vi "PIDController_Calculate_PV.vi"(10 "PV":dbl, 11 "in PID_CONTROLLER":T1={"Kp"=0.0, "Ki"=0.0, "Kd"=0.0, "Period"=0.0, "Max_Integral"=0.0, "Min_Integral"=0.0, "Max_Input"=0.0, "Min_Input"=0.0, "Continuous"=FALSE, "PositionError"=0.0, "VelocityError"=0.0, "PrevError"=0.0, "TotalError"=0.0, "PositionTolerance"=0.0, "VelocityTolerance"=0.0, "SetPoint"=0.0, "Kf"=0.0, "Prev_Deriv"=0.0, "Prev_Deriv 2"=0.0, "DerivativeFilter"=FALSE, "Min_Output"=-9.99e+35, "Max_Output"=9.9e+35, "Prev_F_P"=0.0, "Prev_F_P_2"=0.0, "AntiWindupActive"=FALSE, "Measurement"=0.0} {"Measurement" format="%16_6e"; "Prev_F_P_2" format="%16_6e"; "Prev_F_P" format="%16_6e"; "Max_Output" format="%16_6e"; "Min_Output" format="%16_6e"; "Prev_Deriv 2" format="%16_6e"; "Prev_Deriv" format="%16_6e"; "Kf" format="%16_6e"; "SetPoint" format="%16_6e"; "VelocityTolerance" format="%16_6e"; "PositionTolerance" format="%16_6e"; "TotalError" format="%16_6e"; "PrevError" format="%16_6e"; "VelocityError" format="%16_6e"; "PositionError" format="%16_6e"; "Min_Input" format="%16_6e"; "Max_Input" format="%16_6e"; "Min_Integral" format="%16_6e"; "Max_Integral" format="%16_6e"; "Period" format="%16_6e"; "Kd" format="%16_6e"; "Ki" format="%16_6e"; "Kp" format="%16_6e"}) -> (1 "ControlOutput":dbl, 3 "out PID_CONTROLLER":T1={"Kp"=0.0, "Ki"=0.0, "Kd"=0.0, "Period"=0.0, "Max_Integral"=0.0, "Min_Integral"=0.0, "Max_Input"=0.0, "Min_Input"=0.0, "Continuous"=FALSE, "PositionError"=0.0, "VelocityError"=0.0, "PrevError"=0.0, "TotalError"=0.0, "PositionTolerance"=0.0, "VelocityTolerance"=0.0, "SetPoint"=0.0, "Kf"=0.0, "Prev_Deriv"=0.0, "Prev_Deriv 2"=0.0, "DerivativeFilter"=FALSE, "Min_Output"=-9.99e+35, "Max_Output"=9.9e+35, "Prev_F_P"=0.0, "Prev_F_P_2"=0.0, "AntiWindupActive"=FALSE, "Measurement"=0.0} {"Measurement" format="%16_6e"; "Prev_F_P_2" format="%16_6e"; "Prev_F_P" format="%16_6e"; "Max_Output" format="%16_6e"; "Min_Output" format="%16_6e"; "Prev_Deriv 2" format="%16_6e"; "Prev_Deriv" format="%16_6e"; "Kf" format="%16_6e"; "SetPoint" format="%16_6e"; "VelocityTolerance" format="%16_6e"; "PositionTolerance" format="%16_6e"; "TotalError" format="%16_6e"; "PrevError" format="%16_6e"; "VelocityError" format="%16_6e"; "PositionError" format="%16_6e"; "Min_Input" format="%16_6e"; "Max_Input" format="%16_6e"; "Min_Integral" format="%16_6e"; "Max_Integral" format="%16_6e"; "Period" format="%16_6e"; "Kd" format="%16_6e"; "Ki" format="%16_6e"; "Kp" format="%16_6e"})   [LabVIEW 2019, in "Trajectory_Library.lvlib"]
doc: "Returns the next output of the PID controller. The saved setpoint (SP) in the PID_Controller data structure is used.\n \nInputs:\n - PID_Controller -- PID_Controller data cluster\n - PV-measurement -- The current measurement of the process variable. (PV)\n\nOutputs:\n - PID_Controller -- Updated PID_Controller data cluster\n - CO-ControlOutput -- Controller output (CO)"
uses:
  Trajectory_Library.lvlib
  PID_CONTROLLER.ctl
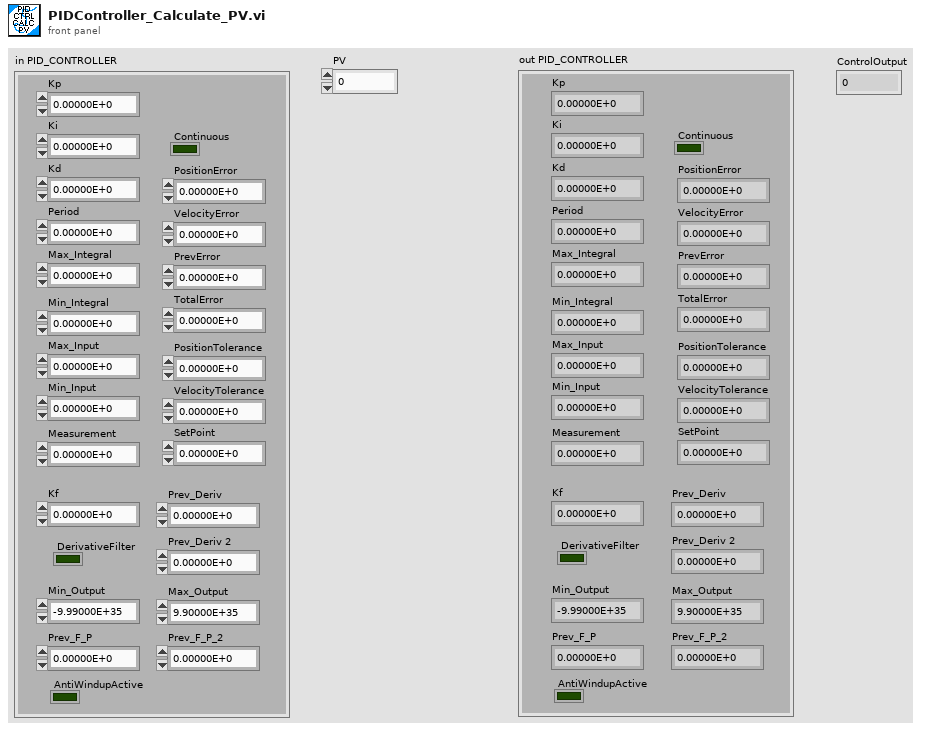
[diagram p1: front panel]
types:
  T1 = typedef "Trajectory_Library.lvlib/PID_CONTROLLER.ctl" = cluster{"Kp":dbl, "Ki":dbl, "Kd":dbl, "Period":dbl, "Max_Integral":dbl, "Min_Integral":dbl, "Max_Input":dbl, "Min_Input":dbl, "Continuous":bool, "PositionError":dbl, "VelocityError":dbl, "PrevError":dbl, "TotalError":dbl, "PositionTolerance":dbl, "VelocityTolerance":dbl, "SetPoint":dbl, "Kf":dbl, "Prev_Deriv":dbl, "Prev_Deriv 2":dbl, "DerivativeFilter":bool, "Min_Output":dbl, "Max_Output":dbl, "Prev_F_P":dbl, "Prev_F_P_2":dbl, "AntiWindupActive":bool, "Measurement":dbl}
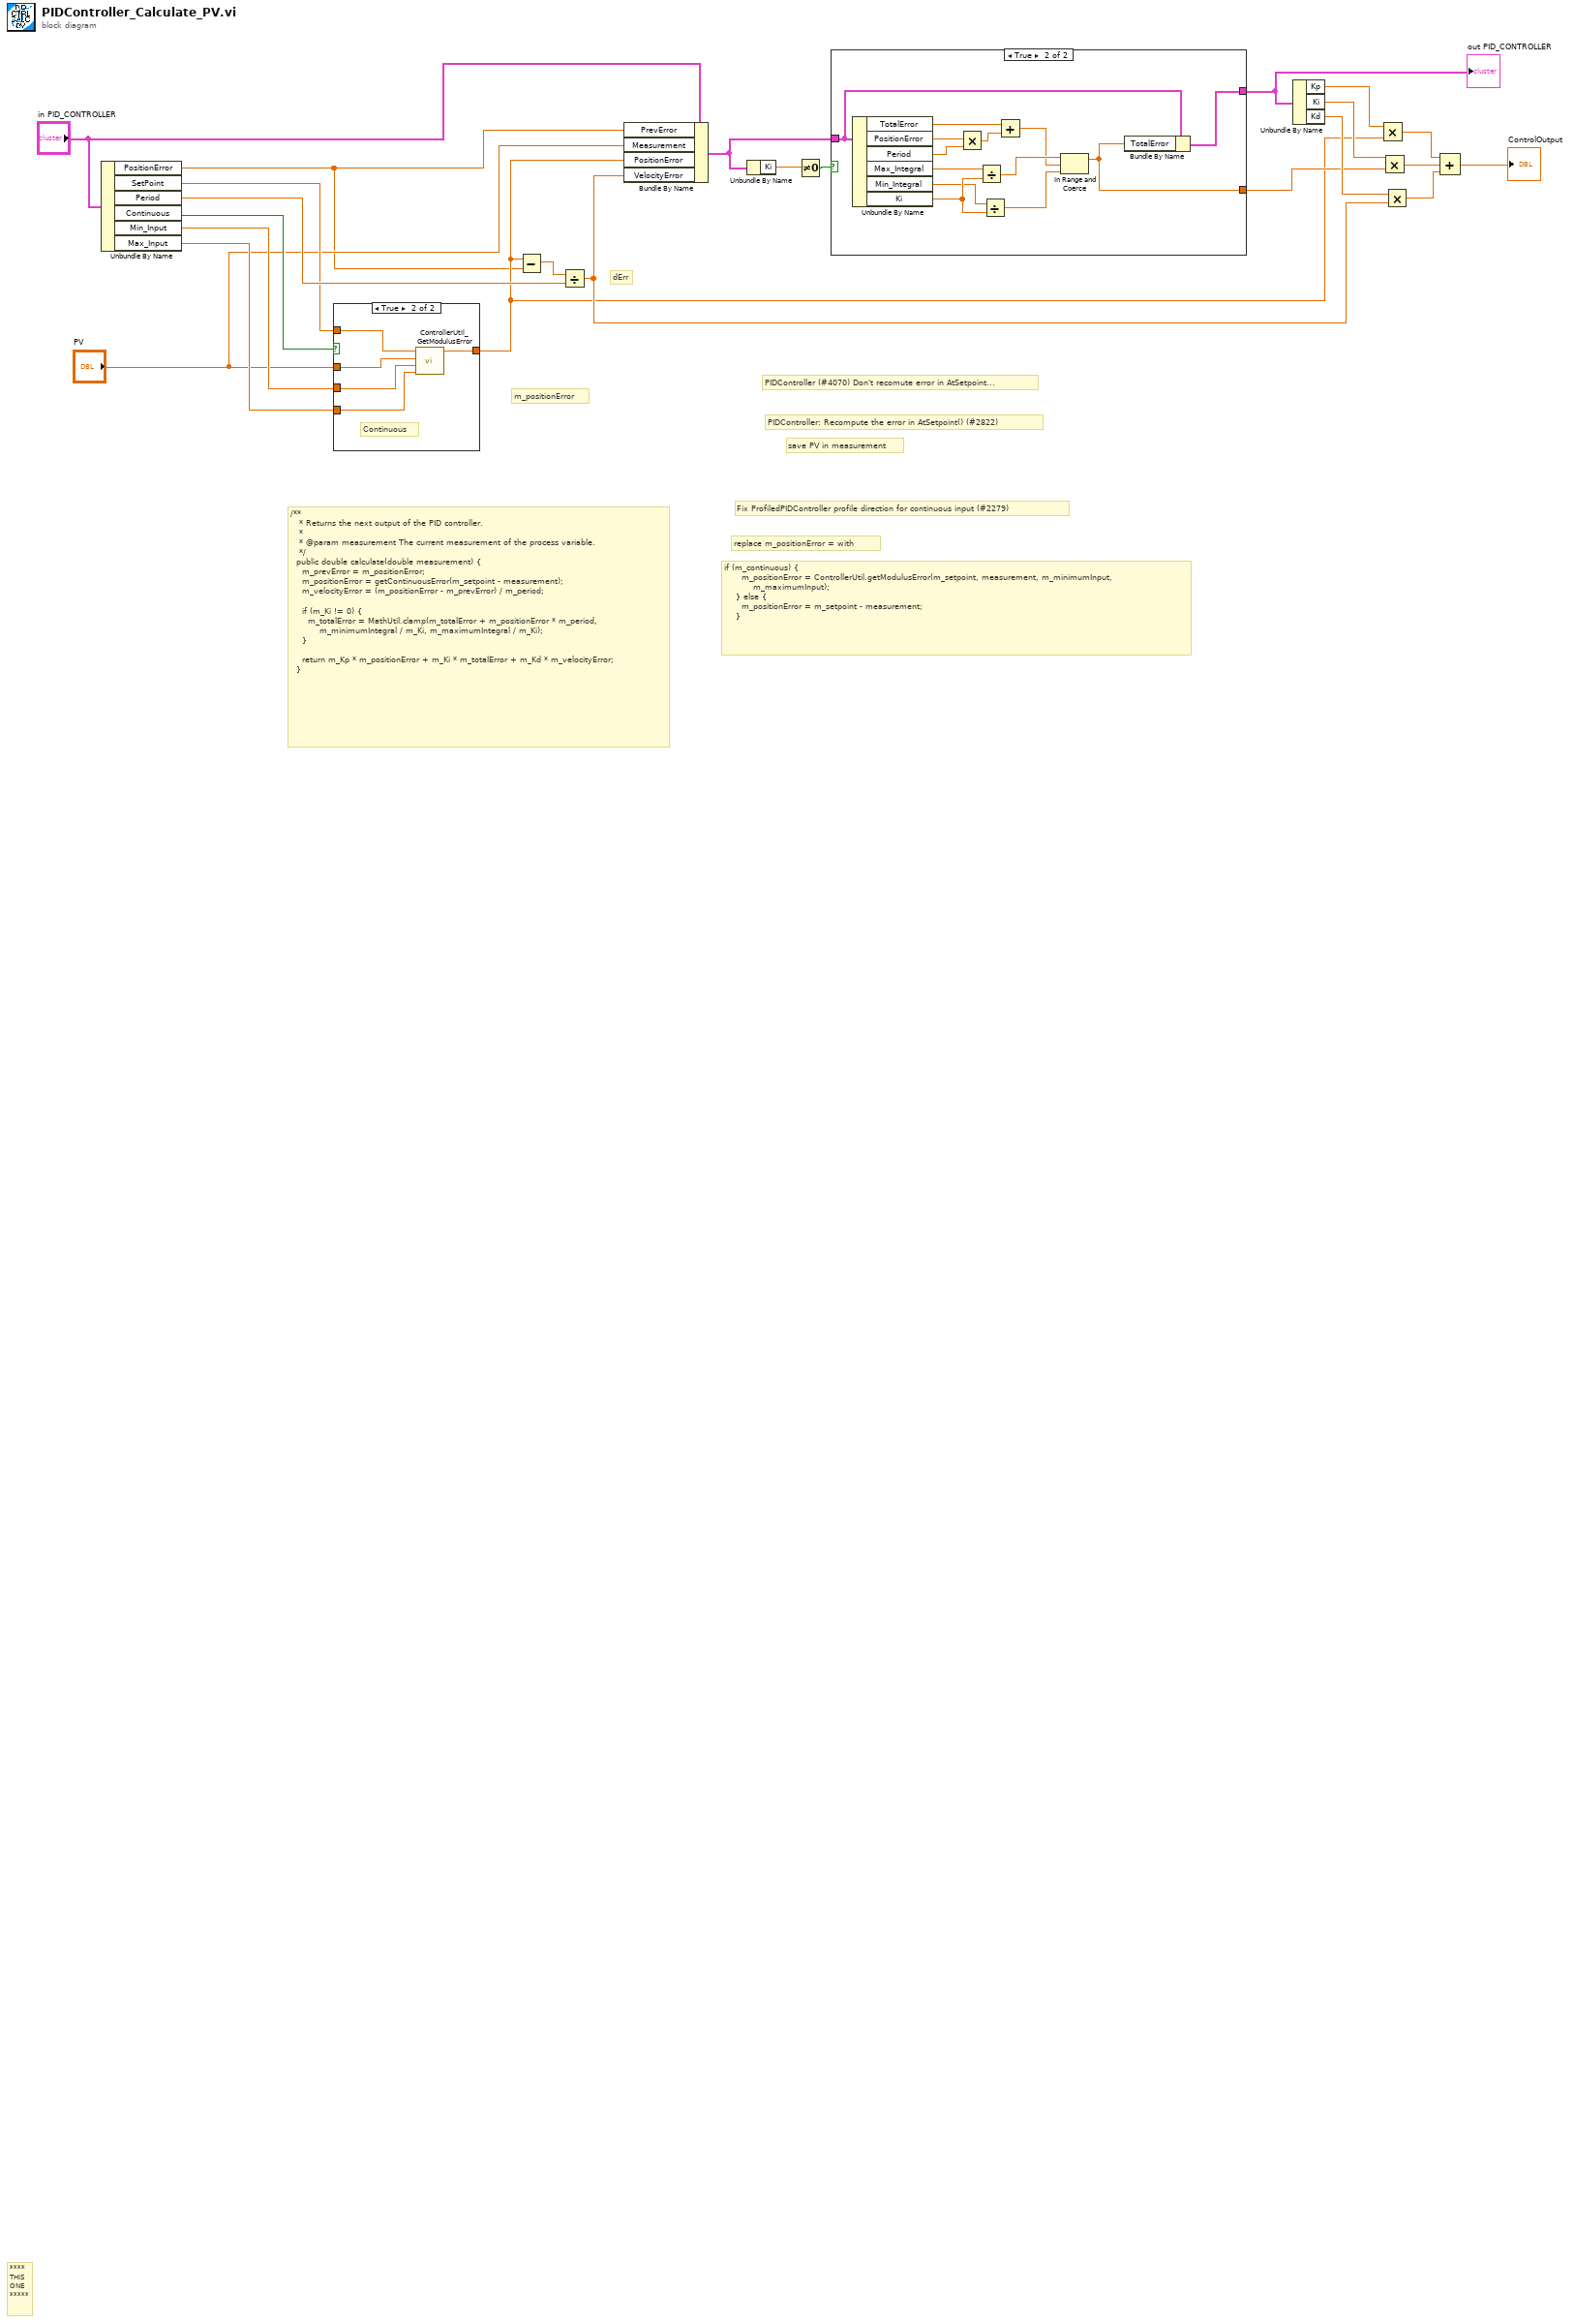
[diagram p0: block diagram]
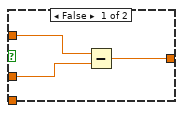
[diagram p2: hidden frame]
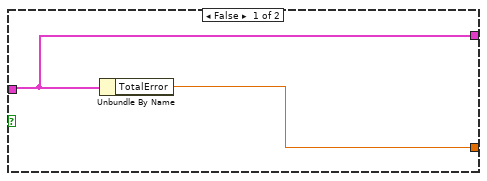
[diagram p3: hidden frame]
diagram:
  # "PIDController (#4070) Don't recomute error in AtSetpoint..."
  # "dErr"
  # "save PV in measurement"
  # "PIDController: Recompute the error in AtSetpoint() (#2822)"
  # "m_positionError"
  # "Fix ProfiledPIDController profile direction for continuous input (#2279)"
  # "replace m_positionError = with"
  # "if (m_continuous) {\n      m_positionError = ControllerUtil.getModulusError(m_setpoint, measurement, m_minimumInput,\n          m_maximumInput);\n    } else {\n      m_positionError = m_setpoint - measurement;\n    }"
  # "/**\n   * Returns the next output of the PID controller.\n   *\n   * @param measurement The current measurement of the process variable.\n   */\n  public double calculate(double measurement) {\n    m_prevError = m_positionError;\n    m_positionError = getContinuousError(m_setpoint - measurement);\n    m_velocityError = (m_positionError - m_prevError) / m_period;\n\n    if (m_Ki != 0) {\n      m_totalError = MathUtil.clamp(m_totalError + m_positionError * m_period,\n          m_minimumIntegral / m_Ki, m_maximumIntegral / m_Ki);\n    }\n\n    return m_Kp * m_positionError + m_Ki * m_totalError + m_Kd * m_velocityError;\n  }"
  # "****\nTHIS\nONE\n*****"
  n1 = Unbundle By Name("in PID_CONTROLLER") -> ("PositionError"=w2:dbl, "SetPoint"=w8:dbl, "Period"=w22:dbl, "Continuous"=w9:bool, "Min_Input"=w6:dbl, "Max_Input"=w5:dbl)
  n2 = case shown="True" w9 {
    tunnel: w8 -> [w26 w31]
    tunnel: "PV" -> [w25 w30]
    tunnel: [w24 w27] -> w7
    tunnel: w6 -> [_ w29]
    tunnel: w5 -> [_ w28]
    frame False {
      n3 = Subtract(x=w26, y=w25) -> (x-y=w24:dbl)
    }
    frame True {
      # "Continuous"
      n4 = call "ControllerUtil_GetModulusError.vi"("Maximum_Input"=w28, "Minimum_Input"=w29, "Measurerment(PV)"=w30, "Reference(SP)"=w31) -> ("Error"=w27:dbl)  [unwired: 7 in]
    }
  }
  n5 = Subtract(x=w7, y=w2) -> (x-y=w23:dbl)
  n6 = Divide(x=w23, y=w22) -> (x/y=w10:dbl)
  n7 = Bundle By Name(cluster="in PID_CONTROLLER", "PrevError"=w2, "Measurement"="PV", "PositionError"=w7, "VelocityError"=w10) -> (w3:T1)
  n8 = Unbundle By Name(w3) -> ("Ki"=w21:dbl)
  n9 = Not Equal To 0?(x=w21) -> (x != 0?=w20:bool)
  n10 = case shown="True" w20 {
    tunnel: w3 -> [w32 w36]
    tunnel: [w32 w35] -> w13
    tunnel: [w33 w34] -> w11
    frame False {
      n11 = Unbundle By Name(w32) -> ("TotalError"=w33:dbl)
    }
    frame True {
      n12 = Unbundle By Name(w36) -> ("TotalError"=w45:dbl, "PositionError"=w44:dbl, "Period"=w43:dbl, "Max_Integral"=w41:dbl, "Min_Integral"=w40:dbl, "Ki"=w42:dbl)
      n13 = Multiply(x=w44, y=w43) -> (x*y=w46:dbl)
      n14 = Divide(x=w41, y=w42) -> (x/y=w39:dbl)
      n15 = Divide(x=w40, y=w42) -> (x/y=w38:dbl)
      n16 = Add(x=w45, y=w46) -> (x+y=w37:dbl)
      n17 = In Range and Coerce(upper limit=w39, x=w37, lower limit=w38) -> (coerced(x)=w34:dbl)  [unwired: 1 out]
      n18 = Bundle By Name(cluster=w36, "TotalError"=w34) -> (w35:T1)
    }
  }
  "out PID_CONTROLLER" <- w13
  n19 = Unbundle By Name(w13) -> ("Kp"=w16:dbl, "Ki"=w15:dbl, "Kd"=w14:dbl)
  n20 = Multiply(x=w16, y=w7) -> (x*y=w19:dbl)
  n21 = Multiply(x=w15, y=w11) -> (x*y=w18:dbl)
  n22 = Multiply(x=w14, y=w10) -> (x*y=w17:dbl)
  n23 = Compound Arithmetic op=ADD(w19, w18, w17) -> (→"ControlOutput":dbl)
